vi "asd.vi"() -> ()   [LabVIEW 2016]
panel:
  out "Waveform Chart 2":dbl(graph)
  out "Waveform Chart":dbl(graph)
  in  "stop":bool
  out "md":dbl(knob) scale=-100.0..100.0
  in  "angulo":dbl(slide) scale=0.0..100.0
  out "mi":dbl(knob) scale=-100.0..100.0
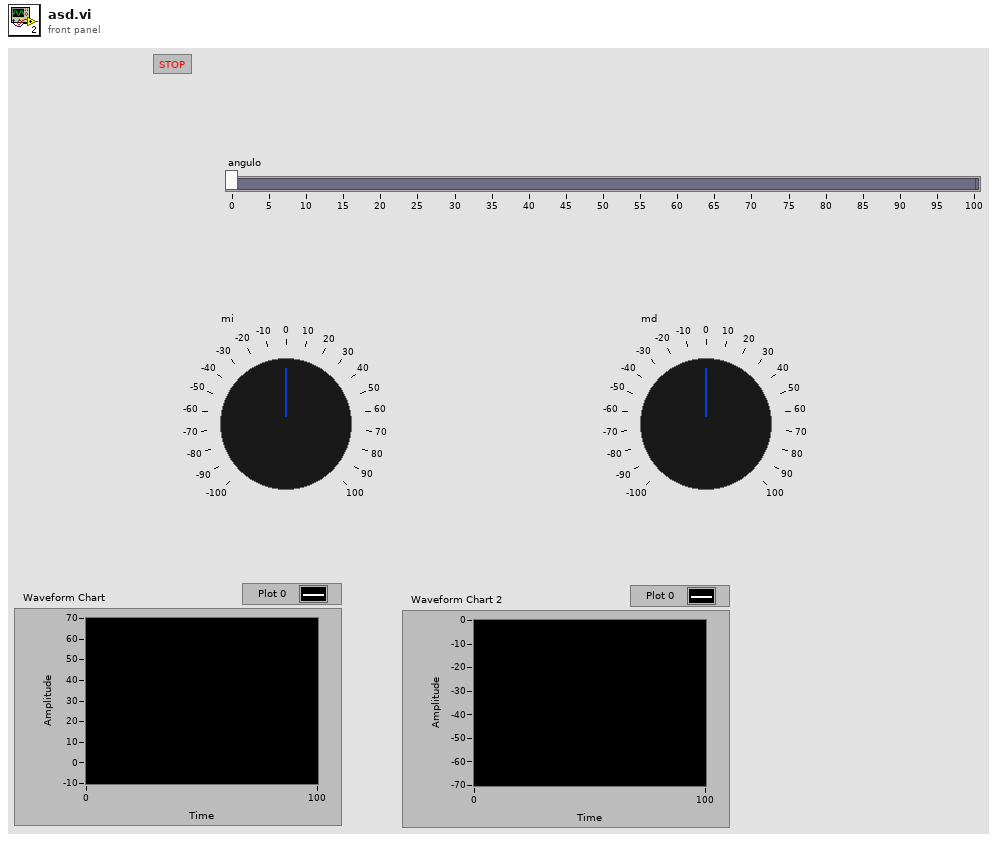
[diagram p1: front panel]
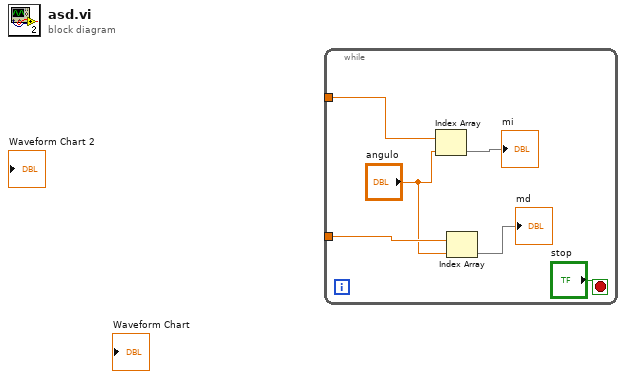
[diagram p0: block diagram]
diagram:
  n1 = while {
    tunnel: [w8] -> w2
    tunnel: [w7] -> w1
    stop <- "stop" stop-if-true
    n2 = Index Array(array=w8, index="angulo") -> (element=→"mi")
    n3 = Index Array(array=w7, index="angulo") -> (element=→"md")
  }
